vi "Get_start_end_ind.vi"(0 "Set_of_Cycles":T1(array[cluster]) {"End_Wait, s" step=1; "N_sweeps" min=0 step=1; "T_sweep, s" min=0.0 step=0.001 format="%#_6f"; "N_steps" min=0 step=1; "fm, kHz" step=1.0; "f0, MHz" min=0.0 step=0.001 format="%#_6f"}) -> (1 "start_ind":i32, 2 "end_ind":i32)   [LabVIEW 2019]
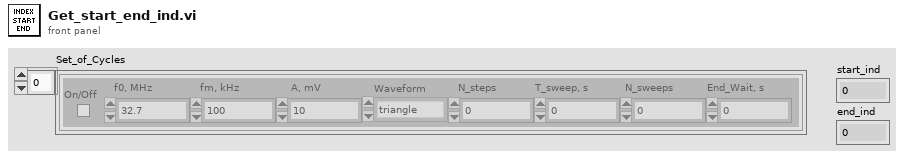
[diagram p1: front panel]
types:
  T1 = cluster{"On/Off":bool, "f0, MHz":dbl, "fm, kHz":dbl, "A, mV":dbl, "Waveform":enum16{"triangle", "saw_direct", "saw_invert", "sine"}, "N_steps":i32, "T_sweep, s":dbl, "N_sweeps":i32, "End_Wait, s":u32}[]
  T2 = cluster{"On/Off":bool, "f0, MHz":dbl, "fm, kHz":dbl, "A, mV":dbl, "Waveform":enum16{"triangle", "saw_direct", "saw_invert", "sine"}, "N_steps":i32, "T_sweep, s":dbl, "N_sweeps":i32, "End_Wait, s":u32}
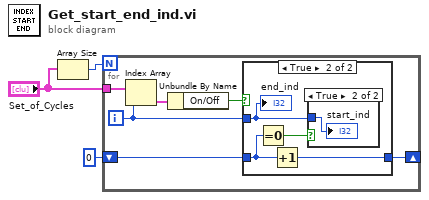
[diagram p0: block diagram]
diagram:
  n1 = Array Size(array="Set_of_Cycles") -> (size(s)=w3:i32)
  n2 = for {
    N: w3 -> [_]
    tunnel: "Set_of_Cycles" -> [w8]
    shift-right: [w5] -> _
    shift-left: 0 -> [w4]
    i -> [w6]
    n3 = Index Array(array=w8, index=w6) -> (element=w9:T2)
    n4 = Unbundle By Name(w9) -> ("On/Off"=w7:bool)
    n5 = case shown="True" w7 {
      tunnel: w6 -> [_ w11]
      tunnel: [w10 w14] -> w5
      tunnel: w4 -> [w10 w12]
      frame False {
      }
      frame True {
        n6 = Equal To 0?(x=w12) -> (x = 0?=w13:bool)
        n7 = Increment(x=w12) -> (x+1=w14:i32)
        n8 = case shown="True" w13 {
          tunnel: w11 -> [_ w15]
          frame False {
          }
          frame True {
            "start_ind" <- w15
          }
        }
        "end_ind" <- w11
      }
    }
  }
